vi "Read Process Step.vi"(7 "Item":T1=enum."sheet heating time", 8 "error in (no error)":errorcluster, 11 "Process Settings in":refnum<class "Process Settings.lvclass">) -> (0 "error out":errorcluster, 1 "Units":T2, 2 "Value":dbl, 3 "Process Settings out":refnum<class "Process Settings.lvclass">)   [LabVIEW 2017, in "Process Settings.lvclass"]
uses:
  Process Settings.lvclass
  Type Defs/Units.ctl
  Type Defs/Item.ctl
  Process Settings.lvclass/Process Settings.ctl
  Accessors/Read Process Step Configs.vi
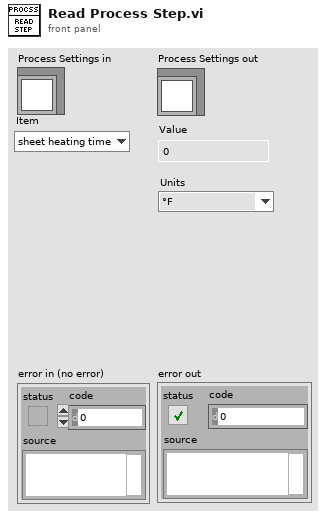
[diagram p1: front panel]
types:
  T1 = typedef "Process Settings.lvclass/Item.ctl" = enum16{"", "sheet temperature setpoint", "sheet heating time", "chamber pressure", "saturation time"}
  T2 = typedef "Process Settings.lvclass/Units.ctl" = enum16{"°F", "°C", "Seconds", "Minutes", "PSIA"}
  T3 = typedef "Process Settings.lvclass/Process Step Description.ctl" = cluster{"Item":T1, "Value":dbl, "Units":T2}
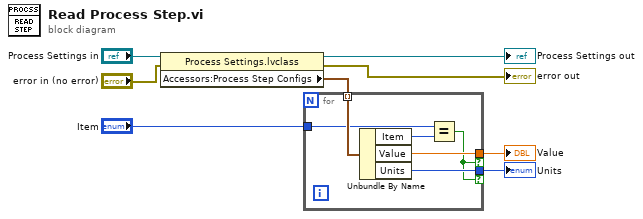
[diagram p0: block diagram]
diagram:
  n1 = property class="Process Settings.lvclass"(reference="Process Settings in", error in="error in (no error)") -> (reference out=→"Process Settings out":refnum<class "Process Settings.lvclass">, error out=→"error out":errorcluster, "Accessors:Process Step Configs"=w5:T3[])
  n2 = for {
    tunnel: w5 -> [w14] mode=indexing
    tunnel: "Item" -> [w13]
    tunnel: [w11] -> w3 if=w9
    tunnel: [w10] -> w2 if=w9
    n3 = Unbundle By Name(w14) -> ("Item"=w12:T1, "Value"=w11:dbl, "Units"=w10:T2)
    n4 = Equal?(x=w13, y=w12) -> (x = y?=w9:bool)
  }
  "Value" <- w3
  "Units" <- w2
